vi "configmgr-variant-test.vi"(8 "error in (no error)":errorcluster) -> (0 "error out":errorcluster)   [LabVIEW 2013]
uses:
  <vilib>/LabVIEW Open Source Project/Configuration Manager/Cache/ConfigManager.Cache.lvclass
  <vilib>/addons/_JKI Toolkits/Caraya/classes/Test/Test.lvclass
  <vilib>/addons/_JKI Toolkits/Caraya/classes/Assert/Assert.lvclass
  <vilib>/LabVIEW Open Source Project/Configuration Manager/Manager/ConfigManager.lvclass
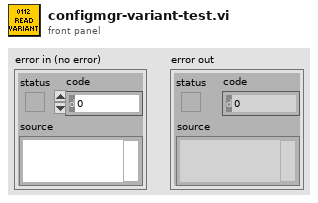
[diagram p1: front panel]
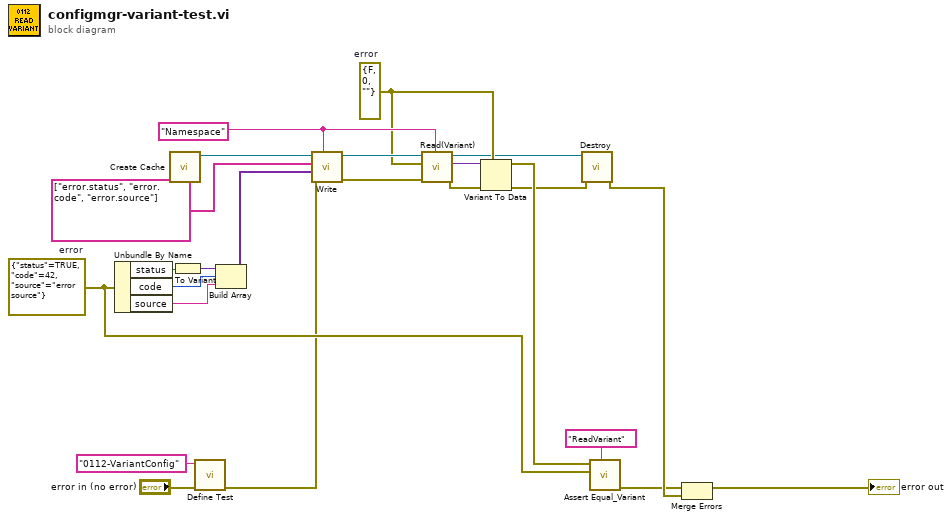
[diagram p0: block diagram]
diagram:
  w11 = errorcluster {"status"=FALSE, "code"=0, "source"=""}  # error
  w7 = errorcluster {"status"=TRUE, "code"=42, "source"="error source"}  # error
  w13 = "Namespace" ("Name")
  n1 = Unbundle By Name(w7) -> ("status"=w19:bool, "code"=w16:i32, "source"=w15:string)
  n2 = call <vilib>:"Create Cache.vi"() -> ("ConfigManager.Cache"=w21:refnum<class "ConfigManager.Cache.lvclass">)  [unwired: 11 in]
  n3 = To Variant(anything=w19) -> (Variant=w18:variant)
  n4 = call <vilib>:"Define Test.vi"("error in (no error)"="error in (no error)", "Label (VI Title)"="0112-VariantConfig") -> ("error out"=w6:errorcluster)  [unwired: 9 in]
  n5 = Build Array(w18, w16, w15) -> (w17:variant[])
  n6 = call <vilib>:"Write.vi"("Qualified Name"=w13, "error in (no error)"=w6, "Values"=w17, "keys"=string[] ["error.status", "error.code", "error.source"], "ConfigManager in"=w21) -> ("error out"=w10:errorcluster, "ConfigManager out"=w14:refnum<class "ConfigManager.Cache.lvclass">)  [unwired: 4 in, 1 out]
  n7 = call <vilib>:"Read(Variant).vi"("Qualified Name"=w13, "error in (no error)"=w10, "Type"=w11, "ConfigManager in"=w14) -> ("error out"=w9:errorcluster, "value"=w12:variant, "ConfigManager out"=w5:refnum<class "ConfigManager.Cache.lvclass">)  [unwired: 3 in, 2 out]
  n8 = Variant To Data(error in=w9, type=w11, Variant=w12) -> (data=w8:errorcluster, error out=w4:errorcluster)
  n9 = call-dynamic "Destroy.vi"("error in (no error)"=w4, "ConfigManager.Cache in"=w5) -> ("error out"=w3:errorcluster)  [unwired: 8 in, 1 out]
  n10 = call <vilib>:"Assert Equal_Variant.vi"("Label"="ReadVariant" ("Label (VI Title)"), "Y"=w7, "X"=w8) -> ("error out"=w2:errorcluster)  [unwired: 8 in]
  n11 = Merge Errors(w2, w3) -> (→"error out":errorcluster)
